vi "漂移计算.vi"(8 "error in (no error)":errorcluster, 11 "input":T1={"索引起始时间"=timestamp(0 s since 1904-01-01), "索引终止时间"=timestamp(0 s since 1904-01-01), "模式"=enum."零点核查", "table"="", "误差"=enum."绝对误差", "技术要求"=0.2, "24H漂移技术要求"=0.05} {"索引终止时间" format="%<%H:%M:%S\n%m/%d/%Y>T"; "索引起始时间" format="%<%H:%M:%S\n%m/%d/%Y>T"}) -> (0 "error out":errorcluster, 2 "列首字符串[]":string[](array[string]), 3 "表格控件":string[][](table))   [LabVIEW 2016, in "数据查询.lvlib"]
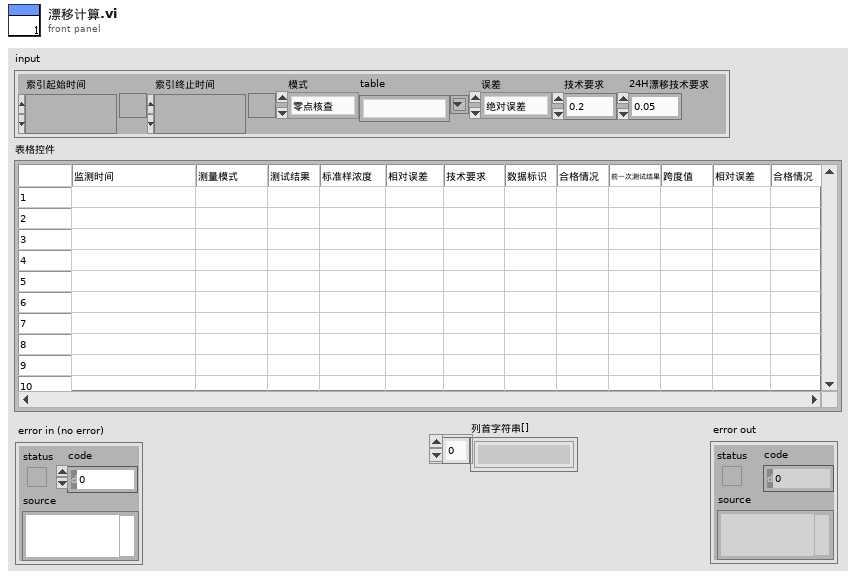
[diagram p1: front panel]
types:
  T1 = cluster{"索引起始时间":timestamp, "索引终止时间":timestamp, "模式":enum16{"零点核查", "跨度核查"}, "table":string, "误差":enum16{"绝对误差", "相对误差"}, "技术要求":sgl, "24H漂移技术要求":sgl}
  T2 = cluster{"索引记录":timestamp, "模式":enum16{"零点核查", "跨度核查"}, "table":string, "误差":enum16{"绝对误差", "相对误差"}, "技术要求":sgl, "24H漂移技术要求":sgl}
  T3 = cluster{"时间":timestamp, "测量模式":string, "值":sgl, "标样参考值":sgl, "数据标识":string, "跨度值":sgl}[]
  T4 = cluster{"时间":timestamp, "测量模式":string, "值":sgl, "标样参考值":sgl, "数据标识":string, "跨度值":sgl}
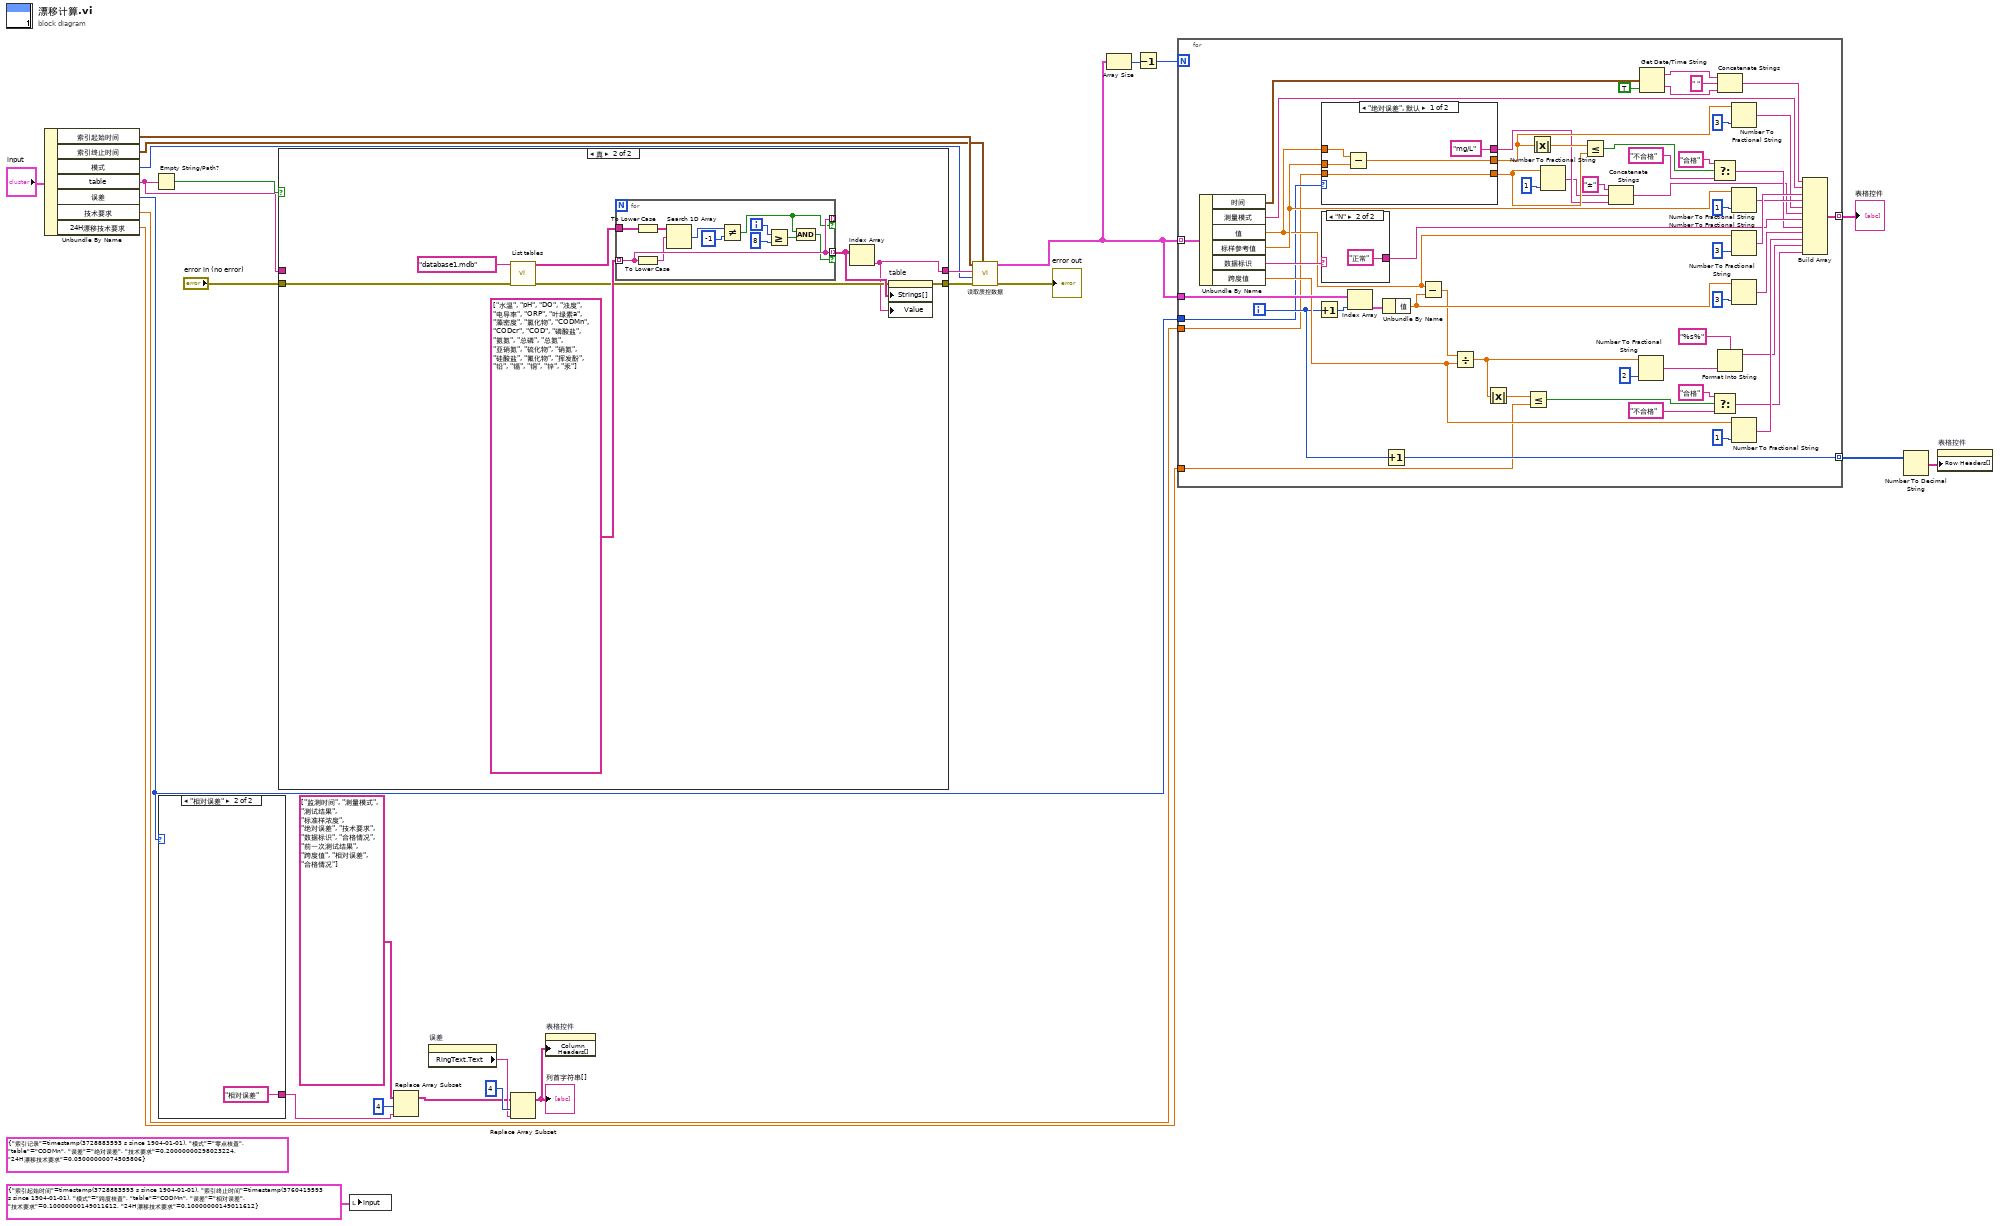
[diagram p0: block diagram]
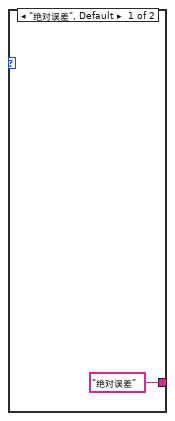
[diagram p2: hidden frame]
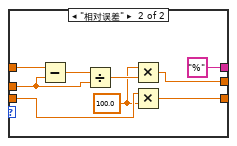
[diagram p4: hidden frame]
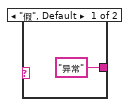
[diagram p5: hidden frame]
diagram:
  (unwired) T2 {"索引记录"=timestamp(3728883593.036628 s since 1904-01-01), "模式"=enum."零点核查", "table"="CODMn", "误差"=enum."绝对误差", "技术要求"=0.2, "24H漂移技术要求"=0.05} ("input")
  n1 = Unbundle By Name("input") -> ("索引起始时间"=w13:timestamp, "索引终止时间"=w8:timestamp, "模式"=w9:enum16{"零点核查", "跨度核查"}, "table"=w12:string, "误差"=w5:enum16{"绝对误差", "相对误差"}, "技术要求"=w11:sgl, "24H漂移技术要求"=w10:sgl)
  n2 = Empty String/Path?(string/path=w12) -> (empty?=w18:bool)
  n3 = case shown="\"相对误差\"" w5 {
    tunnel: ["绝对误差" "相对误差"] -> w3
    frame "绝对误差", Default {
    }
    frame "相对误差" {
    }
  }
  n4 = case shown="真" w18 {
    tunnel: [w31 w34] -> w20
    tunnel: [w30 w33] -> w19
    tunnel: w12 -> [w31 _]
    tunnel: "error in (no error)" -> [w30 w32]
    frame False {
    }
    frame True {
      n5 = call "List tables.vi"("error in (no error)"=w32, "database"="database1.mdb") -> ("error out"=w35:errorcluster, "tables"=w37:string[])  [unwired: 8 in]
      n6 = for {
        tunnel: string[] ["水温", "pH", "DO", "浊度", "电导率", "ORP", "叶绿素a", "藻密度", "氯化物", "CODMn", "CODcr", "COD", "磷酸盐", "氨氮", "总磷", "总氮", "亚硝氮", "硫化物", "硝氮", "硅酸盐", "氟化物", "挥发酚", "铅", "镉", "铜", "锌", "汞"] -> [w47] mode=indexing
        tunnel: w37 -> [w50]
        tunnel: [w47] -> _ mode=indexing if=w42
        tunnel: [w47] -> w36 mode=indexing if=w43
        i -> [w46]
        n7 = To Lower Case(string=w50) -> (all lower case string=w41:string[])
        n8 = To Lower Case(string=w47) -> (all lower case string=w40:string)
        n9 = Search 1D Array(1D array=w41, element=w40) -> (index of element=w49:i32)  [unwired: 1 in]
        n10 = Not Equal?(x=w49, y=-1 ("x")) -> (x != y?=w42:bool)
        n11 = Greater Or Equal?(x=w46, y=8) -> (x >= y?=w44:bool)
        n12 = And(x=w42, y=w44) -> (x .and. y?=w43:bool)
      }
      n13 = Index Array(array=w36) -> (element=w34:string)  [unwired: 1 in]
      n14 = property on="table" class="CmbBox"(error in=w35, "Strings[]"=w36, "Value"=w34) -> (error out=w33:errorcluster)  [unwired: 1 in, 1 out]
    }
  }
  n15 = local write "input"(T1 {"索引起始时间"=timestamp(3728883593.036628 s since 1904-01-01), "索引终止时间"=timestamp(3760419593.036628 s since 1904-01-01), "模式"=enum."跨度核查", "table"="CODMn", "误差"=enum."相对误差", "技术要求"=0.1, "24H漂移技术要求"=0.1} ("input")) -> ()
  n16 = Replace Array Subset(array=string[] ["监测时间", "测量模式", "测试结果", "标准样浓度", "绝对误差", "技术要求", "数据标识", "合格情况", "前一次测试结果", "跨度值", "相对误差", "合格情况"], new element=w3, index=4 ("索引")) -> (w1:string[])
  n17 = property on="误差" class="Enum (严格)"() -> ("RingText.Text"=w15:string)  [unwired: 2 in, 2 out]
  n18 = Replace Array Subset(array=w1, new element=w15, index=4 ("索引")) -> (w6:string[])
  "列首字符串[]" <- w6
  n19 = property on="表格控件" class="Tbl (严格)"("Column Headers[]"=w6) -> ()  [unwired: 2 in, 2 out]
  n20 = call "读取质控数据.vi"("结束索引记录"=w8, "错误输入（无错误）"=w19, "模式"=w9, "table"=w20, "起始索引记录"=w13) -> ("错误输出"=→"error out":errorcluster, "data"=w24:T3)  [unwired: 5 in]
  n21 = Array Size(array=w24) -> (size(s)=w23:i32)
  n22 = Decrement(x=w23) -> (x-1=w22:i32)
  n23 = for {
    N: w22 -> [_]
    tunnel: w24 -> [w106] mode=indexing
    tunnel: [w100] -> w21 mode=indexing
    tunnel: [w97] -> w26 mode=indexing
    tunnel: w24 -> [w84]
    tunnel: w5 -> [w53]
    tunnel: w11 -> [w52]
    tunnel: w10 -> [w51]
    i -> [w66]
    n24 = Unbundle By Name(w106) -> ("时间"=w65:timestamp, "测量模式"=w64:string, "值"=w79:sgl, "标样参考值"=w96:sgl, "数据标识"=w94:string, "跨度值"=w76:sgl)
    n25 = Increment(x=w66) -> (x+1=w83:i32)
    n26 = case shown="\"绝对误差\", 默认" w53 {
      tunnel: w96 -> [w111 w118]
      tunnel: [w110 w113] -> w92
      tunnel: w79 -> [w109 w120]
      tunnel: ["mg/L" "%"] -> w55
      tunnel: w52 -> [w107 w115]
      tunnel: [w107 w114] -> w61
      frame "绝对误差", Default {
        n27 = Subtract(x=w109, y=w111) -> (x-y=w110:sgl)
      }
      frame "相对误差" {
        w112 = sgl 100.0 ("y")
        n28 = Subtract(x=w120, y=w118) -> (x-y=w119:sgl)
        n29 = Divide(x=w119, y=w118) -> (x/y=w117:sgl)
        n30 = Multiply(x=w112, y=w117) -> (x*y=w113:sgl)
        n31 = Multiply(x=w115, y=w112) -> (x*y=w114:sgl)
      }
    }
    n32 = case shown="\"N\"" w94 {
      tunnel: ["异常" ("元素") "正常" ("元素")] -> w93
      frame "假", Default {
      }
      frame "N" {
      }
    }
    n33 = Index Array(array=w84, index=w83) -> (element=w82:T4)
    n34 = Unbundle By Name(w82) -> ("值"=w78:sgl)
    n35 = Increment(x=w66) -> (x+1=w97:i32)
    n36 = Subtract(x=w79, y=w78) -> (x-y=w77:sgl)
    n37 = Divide(x=w77, y=w76) -> (x/y=w72:sgl)
    n38 = Absolute Value(x=w72) -> (abs(x)=w71:sgl)
    n39 = Less Or Equal?(x=w71, y=w51) -> (x <= y?=w69:bool)
    n40 = Absolute Value(x=w92) -> (abs(x)=w91:sgl)
    n41 = Number To Fractional String(number=w61, precision (6)=i16 1 ("精度(6)")) -> (F-format string=w54:string)  [unwired: 2 in]
    n42 = Less Or Equal?(x=w91, y=w61) -> (x <= y?=w90:bool)
    n43 = Concatenate Strings("±", w54, w55) -> (w85:string)
    n44 = Number To Fractional String(number=w72, precision (6)=i16 2 ("精度(6)")) -> (F-format string=w74:string)  [unwired: 2 in]
    n45 = Get Date/Time String(seconds (now)=w65, want seconds? (F)=TRUE ("需要秒？(F)")) -> (date string=w104:string, time string=w98:string)  [unwired: 1 in]
    n46 = Select(t="合格" ("元素"), s=w90, f="不合格" ("元素")) -> (s? t:f=w87:string)
    n47 = Select(t="合格" ("元素"), s=w69, f="不合格" ("元素")) -> (s? t:f=w67:string)
    n48 = Concatenate Strings(w104, " " ("字符串"), w98) -> (w103:string)
    n49 = Format Into String(format string="%s%" ("格式字符串"), w74) -> (resulting string=w73:string)  [unwired: 2 in, 1 out]
    n50 = Number To Fractional String(number=w92, precision (6)=i16 3 ("精度(6)")) -> (F-format string=w95:string)  [unwired: 2 in]
    n51 = Number To Fractional String(number=w96, precision (6)=i16 1 ("精度(6)")) -> (F-format string=w101:string)  [unwired: 2 in]
    n52 = Number To Fractional String(number=w79, precision (6)=i16 3 ("精度(6)")) -> (F-format string=w102:string)  [unwired: 2 in]
    n53 = Number To Fractional String(number=w78, precision (6)=i16 3 ("精度(6)")) -> (F-format string=w81:string)  [unwired: 2 in]
    n54 = Number To Fractional String(number=w76, precision (6)=i16 1 ("精度(6)")) -> (F-format string=w80:string)  [unwired: 2 in]
    n55 = Build Array(w103, w64, w102, w101, w95, w85, w93, w87, w81, w80, w73, w67) -> (w100:string[])
  }
  "表格控件" <- w21
  n56 = Number To Decimal String(number=w26) -> (decimal integer string=w25:string[])  [unwired: 1 in]
  n57 = property on="表格控件" class="Tbl (严格)"("Row Headers[]"=w25) -> ()  [unwired: 2 in, 2 out]
